vi "2D array delete selected columns.vi"(7 "colums to be deleted":i32[](array[numeric]), 11 "input 2d array":dbl[][](array[numeric])) -> (3 "output 2d array":dbl[][](array[numeric]))   [LabVIEW 2019]
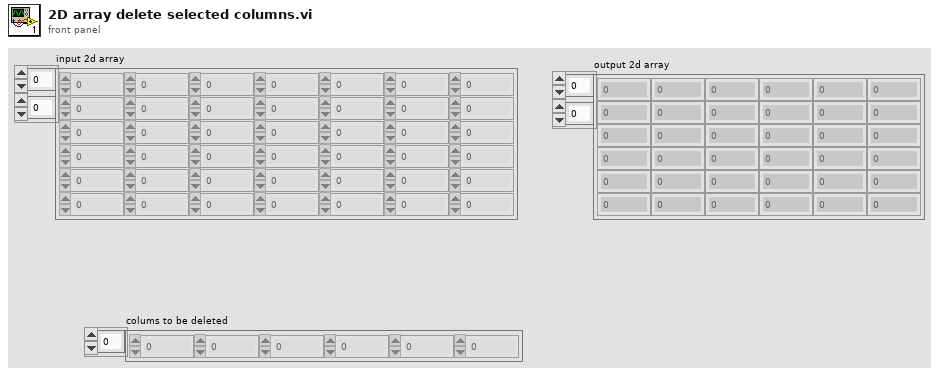
[diagram p1: front panel]
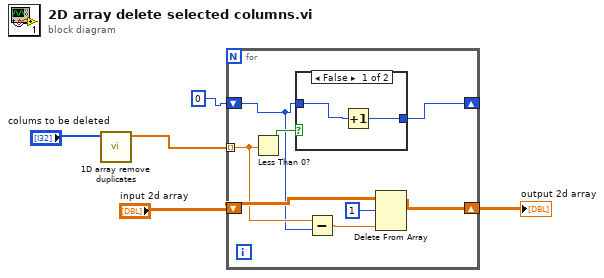
[diagram p0: block diagram]
diagram:
  n1 = call "1D array remove duplicates.vi"("input array"="colums to be deleted") -> ("output array"=w1:dbl[])  [unwired: 10 in]
  n2 = for {
    tunnel: w1 -> [w8] mode=indexing
    shift-right: [w11] -> w3
    shift-left: "input 2d array" -> [w12]
    shift-right: [w9] -> _
    shift-left: 0 ("length") -> [w7]
    n3 = Less Than 0?(x=w8) -> (x < 0?=w10:bool)
    n4 = case shown="False" w10 {
      tunnel: w7 -> [w15 w16]
      tunnel: [w14 w16] -> w9
      frame False {
        n5 = Increment(x=w15) -> (x+1=w14:i32)
      }
      frame True {
      }
    }
    n6 = Subtract(x=w8, y=w7) -> (x-y=w6:dbl)
    n7 = Delete From Array(array=w12, length=1, index (col)=w6) -> (array with subset deleted=w11:dbl[][])  [unwired: 1 in, 1 out]
  }
  "output 2d array" <- w3
